vi "Create TMP File.vi"(3 "PrefixString(\"xxx\")":string="xxx") -> (0 "Last Four":i32 format="%.0x", 1 "Path":path)   [LabVIEW 2011]
uses:
  kernel32.dll
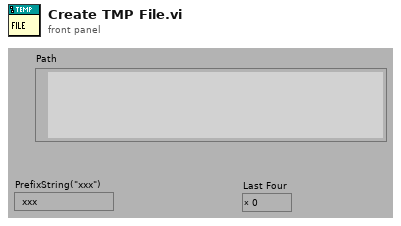
[diagram p1: front panel]
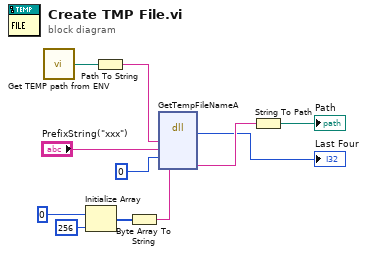
[diagram p0: block diagram]
diagram:
  n1 = call "Get TEMP path from ENV.vi"() -> ("TEMP Path"=w11:path)  [unwired: 5 out]
  n2 = Initialize Array(u8 0, u32 256 ("Dimension Size")) -> (w6:u8[])
  n3 = Path To String(path=w11) -> (string=w10:string)
  n4 = Byte Array To String(unsigned byte array=w6) -> (string=w4:string)
  n5 = dll-call lib="kernel32.dll" fn="GetTempFileNameA"("lpszPath"=w10, "lpPrefixString"="PrefixString(\"xxx\")", "wUnique"=0, "lpTempFileName"=w4) -> (→"Last Four":i32, "lpTempFileName"=w3:string)  [unwired: 6 in, 2 out]
  n6 = String To Path(string=w3) -> (path=→"Path":path)
